vi "NISync_Create.vi"(8 "error in (no error)":errorcluster, 11 "reference in":refnum<class "NISync.lvclass">) -> (0 "error out":errorcluster, 3 "reference out":refnum<class "NISync.lvclass">)   [LabVIEW 2019, in "NISync.lvclass"]
doc: "Constructor."
uses:
  NISync.lvclass
  C:/Program Files/National Instruments/LabVIEW 2019/vi.lib/addons/_AddQ/G#Object/G#Object.lvclass
  C:/Barkhausen mmWave radar/Development/LV/Barkhausen mmWave hardware control/Host/SubVIs/Timing_class/Timing.lvclass
  <vilib>/addons/_AddQ/G#Object/G#Object.lvclass
  Timing_class/Timing.lvclass
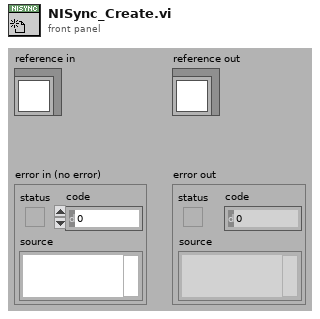
[diagram p1: front panel]
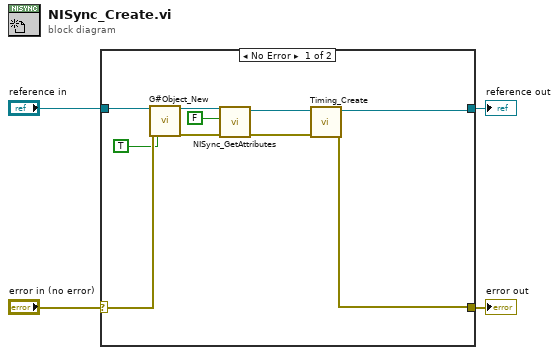
[diagram p0: block diagram]
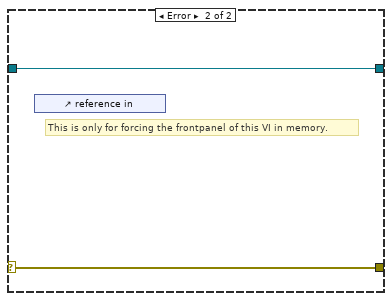
[diagram p2: hidden frame]
diagram:
  n1 = case shown="No Error" "error in (no error)" {
    selector: "error in (no error)" -> [w13 w16]
    tunnel: [w5 w16] -> w3
    tunnel: [w6 w15] -> w1
    tunnel: "reference in" -> [w14 w15]
    frame No Error {
      n2 = call <vilib>:"G#Object_New.vi"("reference in"=w14, "error in (no error)"=w13, "user counter (T)?"=TRUE ("User Counter")) -> ("reference out"=w9:refnum<class "NISync.lvclass">, "error out"=w8:errorcluster)  [unwired: 14 in, 1 out]
      n3 = call "NISync_GetAttributes.vi"("error in (no error)"=w8, "return data? (T)"=FALSE ("return data"), "reference in"=w9) -> ("error out"=w11:errorcluster, "reference out"=w7:refnum<class "NISync.lvclass">)  [unwired: 5 in, 2 out]
      n4 = call "Timing_Create.vi"("error in (no error)"=w11, "reference in"=w7) -> ("error out"=w5:errorcluster, "reference out"=w6:refnum<class "NISync.lvclass">)  [unwired: 8 in]
    }
    frame Error {
      # "This is only for forcing the frontpanel of this VI in memory."
      n5 = control-ref of="reference in"() -> ()  [unwired: 1 out]
    }
  }
  "error out" <- w3
  "reference out" <- w1
